vi "createContext.vi"(8 "error in (no error)":errorcluster, 11 "Boot in":refnum<class "Boot.lvclass">) -> (0 "error out":errorcluster, 2 "Context":refnum<class "Context.lvclass">, 3 "Boot out":refnum<class "Boot.lvclass">)   [LabVIEW 2016, in "Boot.lvclass"]
uses:
  Boot.lvclass
  Context/Context.lvclass
  Context/Context.lvclass/Context.ctl
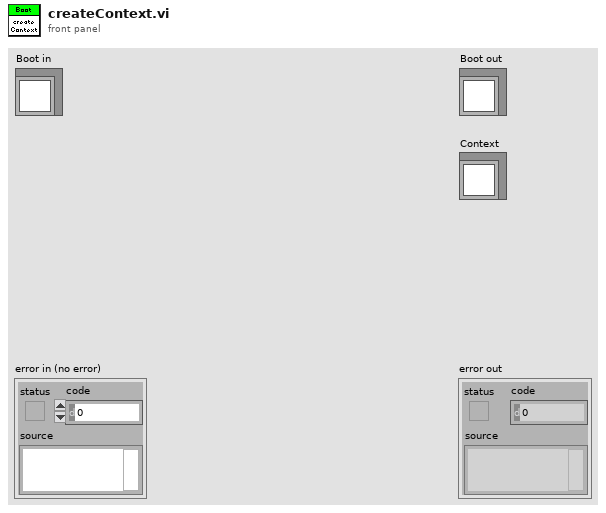
[diagram p1: front panel]
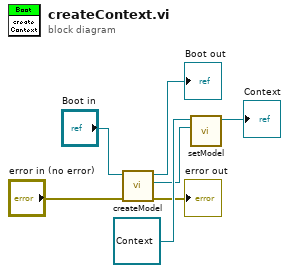
[diagram p0: block diagram]
diagram:
  n1 = call "createModel.vi"("error in (no error)"="error in (no error)", "Boot in"="Boot in") -> ("error out"=→"error out":errorcluster, "Model"=w4:refnum<class "Model.lvclass">, "Boot out"=→"Boot out":refnum<class "Boot.lvclass">)  [unwired: 7 in]
  n2 = call "setModel.vi"("Model"=w4, "Context in"=refnum<class "Context.lvclass"> refnum ("Context.lvclass")) -> ("Context out"=→"Context":refnum<class "Context.lvclass">)  [unwired: 9 in]
